vi "quardrant distribution.vi"(9 "rad":dbl, 10 "input radial point":dbl) -> (0 "quardrant 4":dbl, 1 "quardrant 3":dbl, 2 "quardrant 2":dbl, 3 "quardrant 1":dbl)   [LabVIEW 2017]
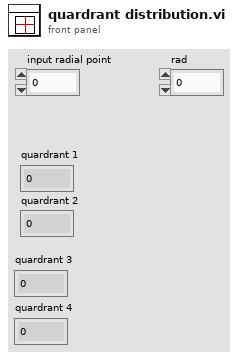
[diagram p1: front panel]
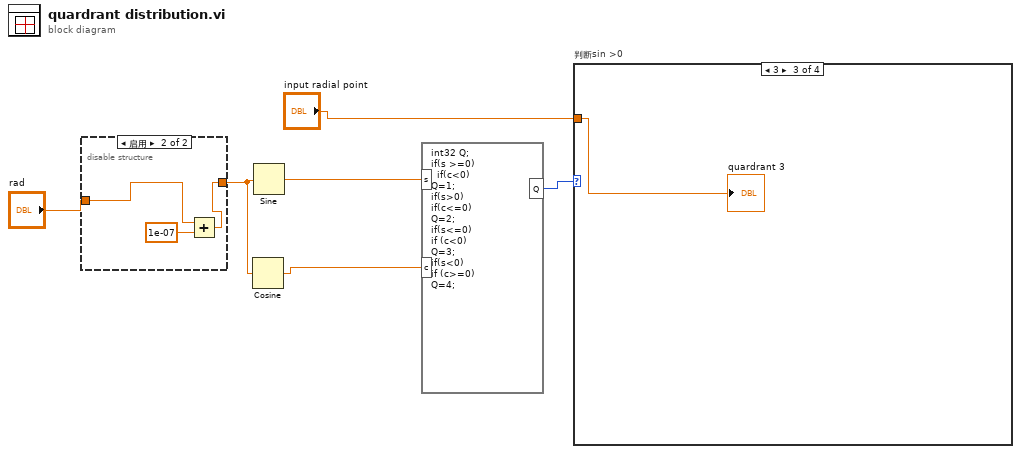
[diagram p0: block diagram]
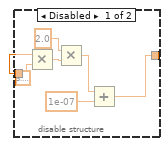
[diagram p2: hidden frame]
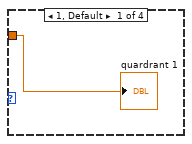
[diagram p3: hidden frame]
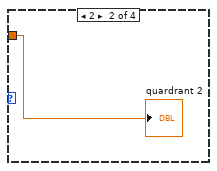
[diagram p4: hidden frame]
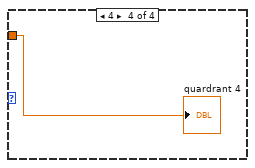
[diagram p5: hidden frame]
diagram:
  n1 = disable-structure shown="启用" {
    disable-tunnel: "rad" -> [w10 w15]
    disable-tunnel: [w7 w14] -> w2
    frame Disabled {
      n2 = Multiply(x=w10, y=3.141592653589793) -> (x*y=w13:dbl)
      n3 = Multiply(x=2.0, y=w13) -> (x*y=w9:dbl)
      n4 = Add(x=w9, y=1e-07) -> (x+y=w7:dbl)
    }
    frame Enabled {
      n5 = Add(x=w15, y=1e-07) -> (x+y=w14:dbl)
    }
  }
  n6 = Cosine(x=w2) -> (cos(x)=w1:dbl)
  n7 = Sine(x=w2) -> (sin(x)=w5:dbl)
  n8 = formula code="int32 Q;\nif(s >=0)\n  if(c<0)\nQ=1;\nif(s>0)\nif(c<=0)\nQ=2;\nif(s<=0)\nif (c<0)\nQ=3;\nif(s<0)\nif (c>=0)\nQ=4;" ("公式节点")("s"=w5, "c"=w1) -> ("Q"=w4:i32)
  n9 = case "判断sin >0" shown="3" w4 {
    tunnel: "input radial point" -> [w17 w18 w19 w20]
    frame 1, Default {
      "quardrant 1" <- w17
    }
    frame 2 {
      "quardrant 2" <- w18
    }
    frame 3 {
      "quardrant 3" <- w19
    }
    frame 4 {
      "quardrant 4" <- w20
    }
  }
